vi "Add Post-process.vi"(5 "Name":string, 6 "Reset":bool, 7 "Subordinate Object":refnum<class "Template Module.lvclass">, 8 "error in (no error)":errorcluster, 9 "Auto launch":bool=TRUE, 10 "Module type":T1, 11 "Monitor-Pulse in":refnum<class "Application Controller.lvclass">) -> (0 "error out":errorcluster, 3 "Monitor-Pulse out":refnum<class "Application Controller.lvclass">)   [LabVIEW 2019, in "Application Controller.lvclass"]
uses:
  Application Controller.lvclass
  Module Types.ctl
  Template Module/Template Module.lvclass
  Application Controller.lvclass/Application Controller.ctl
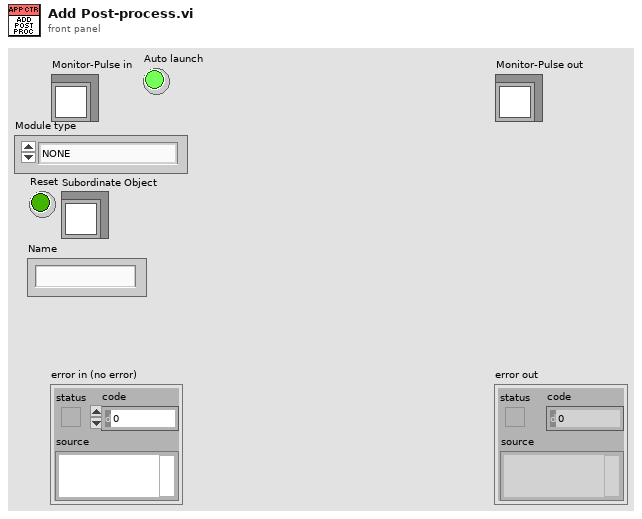
[diagram p1: front panel]
types:
  T1 = typedef "Module Types.ctl" = enum16{"NONE", "NI-DAQmx", "NI-Scope", "Red Pitaya Digitizer", "GaGe", "VISA Device", "Red Pitaya Lockin", "Monitor Controller", "Pulse Controller", "Integrate Pulse", "Lockin Processor", "File converter", "NHMFL Synthesizer", "Micron Hyperion", "Spectrum Recorder", "Resonance Detector", "TCP Communications", "Format Resonances", "Ruby Spectra", "PID Controller", "Quantum Design", "VI Server"}
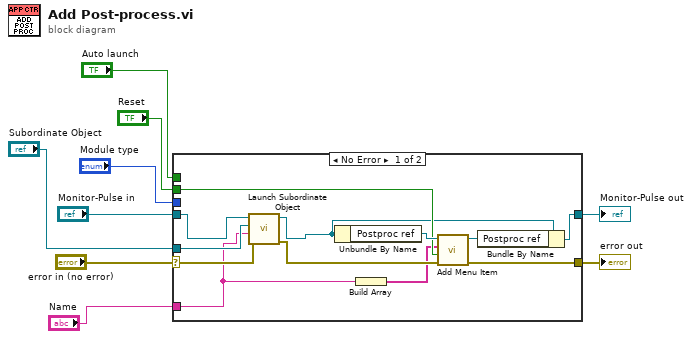
[diagram p0: block diagram]
diagram:
  n1 = case shown="No Error" "error in (no error)" {
    selector: "error in (no error)" -> [w13 w23]
    tunnel: [w17 w23] -> w8
    tunnel: [w19 w22] -> w6
    tunnel: "Monitor-Pulse in" -> [w16 w22]
    tunnel: "Module type" -> [_ _]
    tunnel: "Auto launch" -> [_ _]
    tunnel: "Reset" -> [w20 _]
    tunnel: "Subordinate Object" -> [w14 _]
    tunnel: "Name" -> [w11 _]
    frame No Error {
      n2 = call-dynamic "Launch Subordinate Object.vi"("error in (no error)"=w13, "Name"=w11, "Subordinate Object"=w14, "Measure Object in"=w16) -> ("error out"=w12:errorcluster, "Measure Object out"=w15:refnum<class "Application Controller.lvclass">)  [unwired: 5 in, 1 out]
      n3 = Unbundle By Name(w15) -> ("Postproc ref"=w21:refnum<vi>)
      n4 = Build Array(w11) -> (w10:string[])
      n5 = call "Add Menu Item.vi"("error in (no error)"=w12, "Reset"=w20, "Item Names"=w10, "Queed Listbox ref"=w21) -> ("error out"=w17:errorcluster, "Queed Listbox ref out"=w18:refnum<vi>)  [unwired: 5 in, 1 out]
      n6 = Bundle By Name(cluster=w15, "Postproc ref"=w18) -> (w19:refnum<class "Application Controller.lvclass">)
    }
    frame Error {
    }
  }
  "error out" <- w8
  "Monitor-Pulse out" <- w6
